vi "Detenerse en cierto tiempo.vi"() -> ()   [LabVIEW 2020]
panel:
  in  "stop":bool
  out "Time has Elapsed":bool
  in  "Reset":bool
  in  "Auto Reset":bool=TRUE
  in  "Time Target (s)":dbl=1.0
  in  "millisecond timer value":u32
  out "Alea":dbl
  out "Numeric":i32
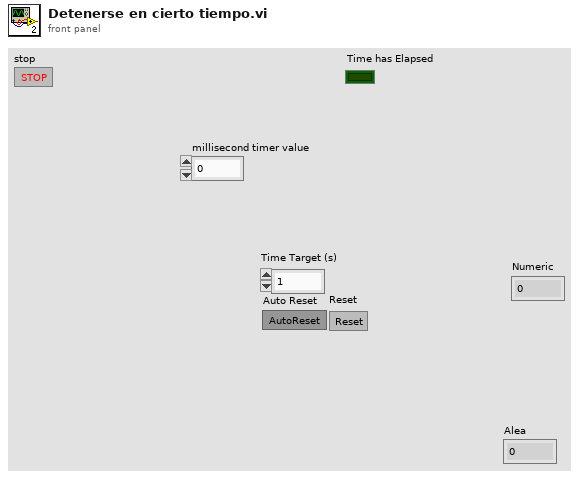
[diagram p1: front panel]
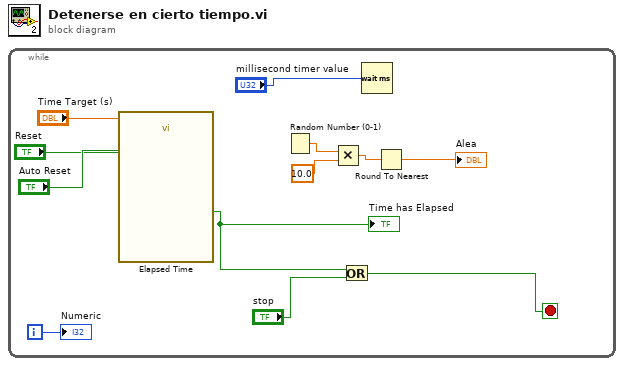
[diagram p0: block diagram]
diagram:
  n1 = while {
    i -> [w12]
    stop <- w1 stop-if-true
    n2 = call "Elapsed Time"("Time Target (s)"="Time Target (s)", "Reset"="Reset", "Auto Reset"="Auto Reset") -> ("Time has Elapsed"=w3:bool)  [unwired: 9 in, 7 out]
    "Time has Elapsed" <- w3
    n3 = Random Number (0-1)() -> (number: 0 to 1=w11:dbl)
    n4 = Multiply(x=w11, y=10.0) -> (x*y=w9:dbl)
    n5 = Or(x=w3, y="stop") -> (x .or. y?=w1:bool)
    n6 = Wait (ms)(milliseconds to wait="millisecond timer value") -> ()  [unwired: 1 out]
    n7 = Round To Nearest(number=w9) -> (nearest integer value=→"Alea":dbl)
    "Numeric" <- w12
  }
